vi "Set Windows Size.vi"(6 "Size":cluster{"cx":i32, "cy":i32}, 8 "error in (no error)":errorcluster, 9 "uFlags":u32(ring)=1 items=["SWP_ASYNCWINDOWPOS"=16384, "SWP_DEFERERASE"=8192, "SWP_DRAWFRAME"=32, "SWP_HIDEWINDOW"=128, "SWP_NOACTIVATE"=16, "SWP_NOCOPYBITS"=256, "SWP_NOMOVE"=2, "SWP_NOOWNERZORDER"=512, "SWP_NOREDRAW"=8, "SWP_NOSENDCHANGING"=1024, "SWP_NOSIZE"=1, "SWP_NOZORDER"=4, "SWP_SHOWWINDOW"=64], 10 "hWndInsertAfter":string(combo), 11 "hWnd":u32) -> (0 "error out":errorcluster, 2 "ok?":bool, 3 "hWnd out":u32)   [LabVIEW 2019, in "Test Bench Tools.lvlib"]
uses:
  Test Bench Tools.lvlib
  user32.dll
panel:
  in  "Position":cluster{"X":i32, "Y":i32}
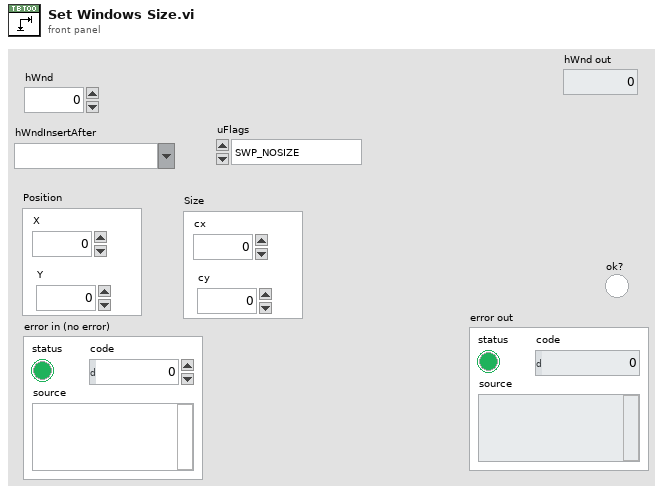
[diagram p1: front panel]
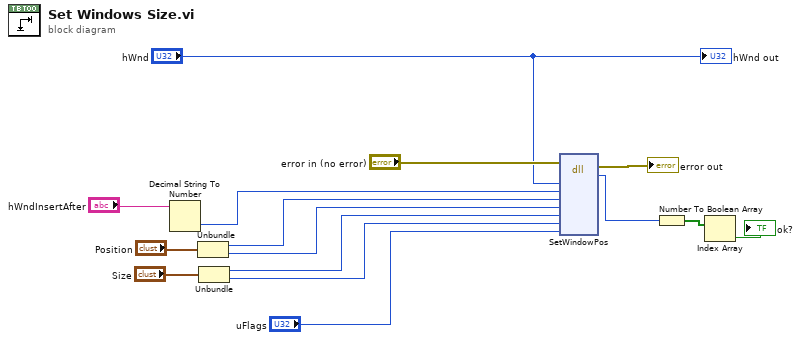
[diagram p0: block diagram]
diagram:
  n1 = Decimal String To Number(string="hWndInsertAfter") -> (number=w6:i32)  [unwired: 2 in, 1 out]
  n2 = Unbundle("Position") -> ("X"=w12:i32, "Y"=w11:i32)
  n3 = Unbundle("Size") -> ("cx"=w9:i32, "cy"=w8:i32)
  n4 = dll-call lib="USER32.DLL" fn="SetWindowPos"(error in="error in (no error)", "hWnd"="hWnd", "hWndInsertAfter"=w6, "left"=w12, "top"=w11, "width"=w9, "height"=w8, "fuFlags"="uFlags") -> (error out=→"error out":errorcluster, "error"=w4:i32)  [unwired: 9 in, 1 out]
  n5 = Number To Boolean Array(number=w4) -> (Boolean array=w3:bool[])
  n6 = Index Array(array=w3) -> (element=→"ok?":bool)  [unwired: 1 in]
  "hWnd out" <- "hWnd"
